vi "XYZStage-Reset axis command (ver 2).vi"(8 "error in (no error)":errorcluster, 10 "XYZ Stage dequeued data":T1={"Command"=enum."Initialize", "Channel"="Z", "X"=0.0, "Y"=0.0, "Z"=0.0, "Speed"=0, "Zero"=FALSE, "Use acknowledgement?"=TRUE} {"Speed" format="Speed= %.0f"; "Z" format="Z= %#_g"; "Y" format="Y= %#_g"; "X" format="X= %#_g"}, 11 "XYZ Stage Control in":refnum<class "XYZ Stage Control.lvclass">) -> (0 "error out":errorcluster, 3 "XYZ Stage Control out":refnum<class "XYZ Stage Control.lvclass">)   [LabVIEW 2020]
uses:
  Typedefs/XYZ stage data.ctl
  Typedefs/XYZ stage states.ctl
  Typedefs/XYZ channel ring.ctl
  XYZ Stage Control/XYZ Stage Control.lvclass
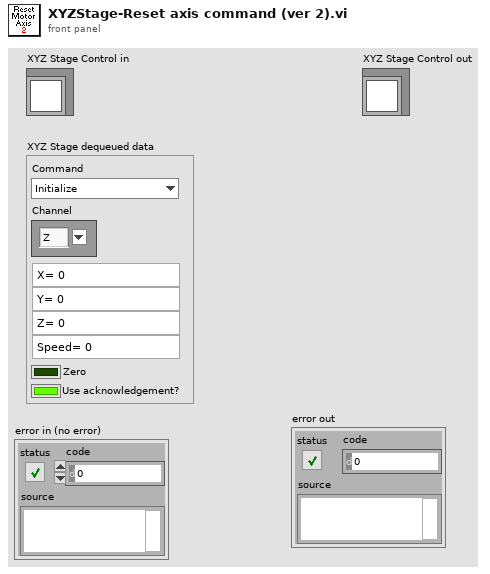
[diagram p1: front panel]
types:
  T1 = typedef "XYZ stage data.ctl" = cluster{"Command":T2, "Channel":T3, "X":sgl, "Y":sgl, "Z":sgl, "Speed":i32, "Zero":bool, "Use acknowledgement?":bool}
  T2 = typedef "XYZ stage states.ctl" = enum16{"Dequeue", "Initialize", "Read Position", "Read Speed Setting", "Move", "Set Max Speed", "Reset Axis", "Stop all movement"}
  T3 = typedef "XYZ channel ring.ctl" = string
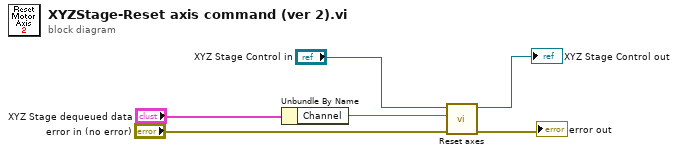
[diagram p0: block diagram]
diagram:
  n1 = Unbundle By Name("XYZ Stage dequeued data") -> ("Channel"=w5:T3)
  n2 = call-dynamic "Reset axes.vi"("error in (no error)"="error in (no error)", "Channel"=w5, "XYZ Stage Control in"="XYZ Stage Control in") -> ("error out"=→"error out":errorcluster, "XYZ Stage Control out"=→"XYZ Stage Control out":refnum<class "XYZ Stage Control.lvclass">)  [unwired: 7 in]
